vi "Test_exe.vi"() -> ()   [LabVIEW 2018]
panel:
  out "Numeric":i32
  in  "Stop":bool
  in  "File Path":path
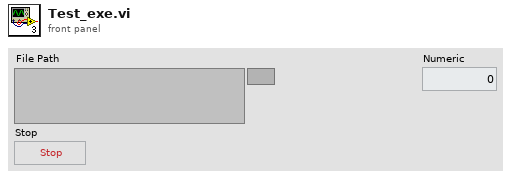
[diagram p1: front panel]
types:
  T1 = typedef "IMAQ Image.ctl" = refnum<image>
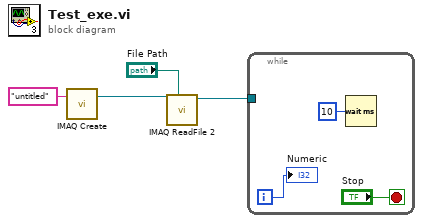
[diagram p0: block diagram]
diagram:
  n1 = call "IMAQ Create"("Image Name"="untitled") -> ("New Image"=w3:T1)  [unwired: 4 in, 1 out]
  n2 = call "IMAQ ReadFile 2"("File Path"="File Path", "Image"=w3) -> ("Image Out"=w1:T1)  [unwired: 5 in, 4 out]
  n3 = while {
    tunnel: w1 -> [_]
    i -> [w6]
    stop <- "Stop" stop-if-true
    n4 = Wait (ms)(milliseconds to wait=u32 10) -> ()  [unwired: 1 out]
    "Numeric" <- w6
  }
